vi "saveDataNode.vi"(8 "error in (no error)":errorcluster, 9 "indent":i32, 10 "XML Refnum in":refnum<file>, 11 "xceDataNode in":refnum<class "xceDataNode.lvclass">) -> (0 "error out":errorcluster, 2 "XML Refnum out":refnum<file>, 3 "xceDataNode out":refnum<class "xceDataNode.lvclass">)   [LabVIEW 2013, in "xceDataNode.lvclass"]
doc: "Saves the tree data structure node to an XML formatted file."
uses:
  xceDataNode.lvclass
  xceNode/xceNode.lvclass
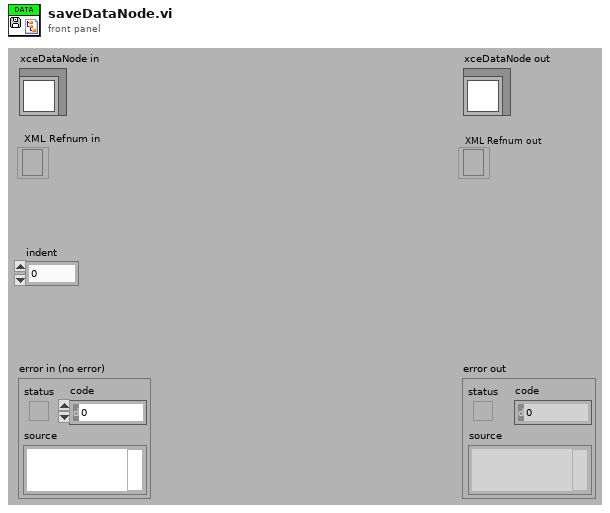
[diagram p1: front panel]
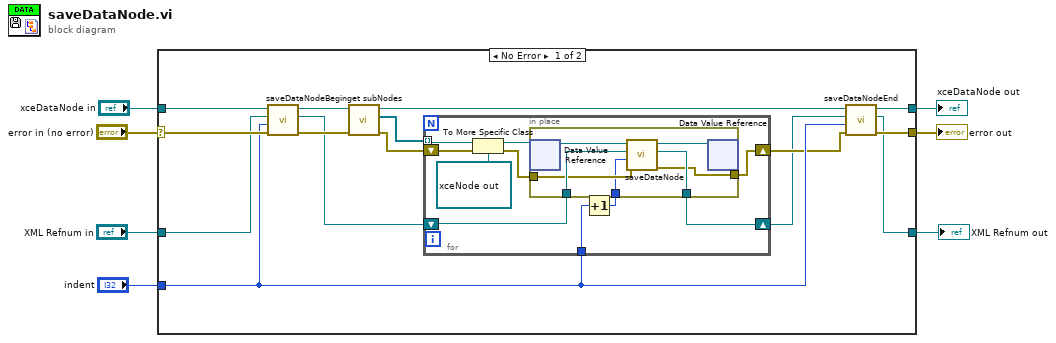
[diagram p0: block diagram]
diagram:
  n1 = case shown="No Error" "error in (no error)" {
    selector: "error in (no error)" -> [w19 w42]
    tunnel: [w10 w42] -> w6
    tunnel: [w13 w41] -> w4
    tunnel: "xceDataNode in" -> [w21 w41]
    tunnel: "XML Refnum in" -> [w18 w40]
    tunnel: "indent" -> [w12 _]
    tunnel: [w9 w40] -> w1
    frame No Error {
      n2 = call-dynamic "saveDataNodeBegin.vi"("error in (no error)"=w19, "indent"=w12, "XML Refnum in"=w18, "xceDataNode in"=w21) -> ("error out"=w17:errorcluster, "XML Refnum out"=w15:refnum<file>, "xceDataNode out"=w20:refnum<class "xceDataNode.lvclass">)  [unwired: 5 in]
      n3 = call "get subNodes.vi"("error in (no error)"=w17, "xceNode in"=w20) -> ("error out"=w16:errorcluster, "subNodes[]*"=w22:refnum<data-value>[], "xceNode out"=w14:refnum<class "xceDataNode.lvclass">)  [unwired: 7 in]
      n4 = for {
        tunnel: w22 -> [w32] mode=indexing
        shift-right: [w27] -> w11
        shift-left: w16 -> [w31]
        tunnel: w12 -> [w24]
        shift-right: [w23] -> w8
        shift-left: w15 -> [w26]
        n5 = To More Specific Class(target class=refnum<data-value> refnum ("data value reference"), reference=w32, error in=w31) -> (specific class reference=w29:refnum<data-value>, error out=w28:errorcluster)
        n6 = Increment(x=w24) -> (x+1=w25:i32)
        n7 = in-place {
          in-place-border: w28 -> [w36]
          in-place-border: [w34] -> w27
          in-place-border: w26 -> [w37]
          in-place-border: [w35] -> w23
          in-place-border: w25 -> [w33]
          n8 = in-place-dvr #1(w29) -> (w38:refnum<class "xceDataNode.lvclass">)  [unwired: 1 out]
          n9 = call "saveDataNode.vi"("error in (no error)"=w36, "indent"=w33, "XML Refnum in"=w37, "xceDataNode in"=w38) -> ("error out"=w34:errorcluster, "XML Refnum out"=w35:refnum<file>, "xceDataNode out"=w39:refnum<class "xceDataNode.lvclass">)  [unwired: 5 in]
          n10 = in-place-dvr #1(w39) -> ()  [unwired: 2 out]
        }
      }
      n11 = call-dynamic "saveDataNodeEnd.vi"("error in (no error)"=w11, "indent"=w12, "XML Refnum in"=w8, "xceDataNode in"=w14) -> ("error out"=w10:errorcluster, "XML Refnum out"=w9:refnum<file>, "xceDataNode out"=w13:refnum<class "xceDataNode.lvclass">)  [unwired: 5 in]
    }
    frame Error {
    }
  }
  "error out" <- w6
  "xceDataNode out" <- w4
  "XML Refnum out" <- w1
